vi "Buffer eq termico.vi"(8 "dt":dbl, 9 "time":dbl, 10 "prova in corso?":bool, 11 "Tempo valutazione":dbl) -> (2 "Array dt":dbl[](array[numeric]), 3 "Array time":dbl[](array[numeric]))   [LabVIEW 2019]
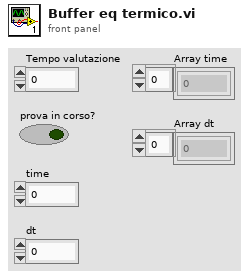
[diagram p1: front panel]
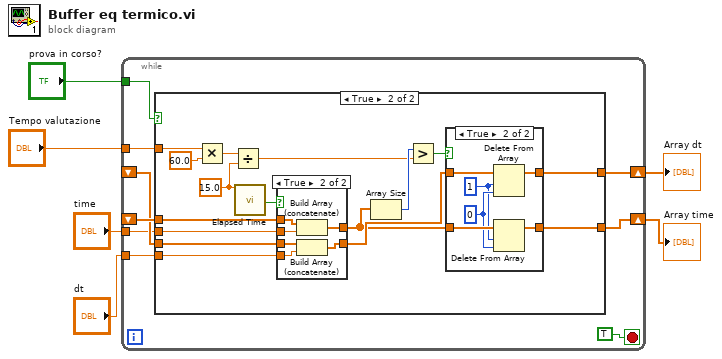
[diagram p0: block diagram]
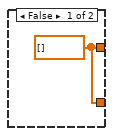
[diagram p2: hidden frame]
diagram:
  n1 = while {
    shift-right: [w14] -> w3
    shift-left: _ -> [w15]
    shift-right: [w11] -> w1
    shift-left: _ -> [w12]
    tunnel: "time" -> [w10]
    tunnel: "dt" -> [w9]
    tunnel: "prova in corso?" -> [w8]
    tunnel: "Tempo valutazione" -> [w7]
    stop <- TRUE stop-if-true
    n2 = case shown="True" w8 {
      tunnel: w15 -> [_ w32]
      tunnel: [w16 w21] -> w14
      tunnel: w12 -> [_ w31]
      tunnel: [w16 w19] -> w11
      tunnel: w10 -> [_ w29]
      tunnel: w9 -> [_ w28]
      tunnel: w7 -> [_ w17]
      frame False {
        w16 = dbl[] []
      }
      frame True {
        w25 = 15.0 ("Time Target (s)")
        n3 = Multiply(x=w17, y=60.0) -> (x*y=w27:dbl)
        n4 = Divide(x=w27, y=w25) -> (x/y=w23:dbl)
        n5 = call "Elapsed Time"("Time Target (s)"=w25) -> ("Time has Elapsed"=w30:bool)  [unwired: 11 in, 7 out]
        n6 = case shown="True" w30 {
          tunnel: w32 -> [w42 w48]
          tunnel: [w42 w47] -> w18
          tunnel: w31 -> [w41 w45]
          tunnel: [w41 w43] -> w20
          tunnel: w29 -> [_ w46]
          tunnel: w28 -> [_ w44]
          frame False {
          }
          frame True {
            n7 = Build Array (concatenate)(w48, w46) -> (w47:dbl[])
            n8 = Build Array (concatenate)(w45, w44) -> (w43:dbl[])
          }
        }
        n9 = Array Size(array=w18) -> (size(s)=w24:i32)
        n10 = Greater?(x=w24, y=w23) -> (0:w22:bool)
        n11 = case shown="True" w22 {
          tunnel: w18 -> [w34 w40]
          tunnel: [w34 w39] -> w21
          tunnel: w20 -> [w33 w38]
          tunnel: [w33 w37] -> w19
          frame False {
          }
          frame True {
            w35 = 1 ("index")
            w36 = 0 ("index")
            n12 = Delete From Array(array=w38, length=w35, index=w36) -> (array with subset deleted=w37:dbl[])  [unwired: 1 out]
            n13 = Delete From Array(array=w40, length=w35, index=w36) -> (array with subset deleted=w39:dbl[])  [unwired: 1 out]
          }
        }
      }
    }
  }
  "Array time" <- w3
  "Array dt" <- w1
